vi "NAVX.vi"() -> ()   [LabVIEW 2018]
uses:
  <vilib>/Studica/Studica Toolkit/Background/I2C Channel.ctl
  <vilib>/Studica/Studica Toolkit/NavX/TypeDefs/Flags/Z900_navX_Flags_OpStatusTypeDef.ctl
  <vilib>/Studica/Studica Toolkit/NavX/TypeDefs/Flags/Z900_navX_Flags_CalibrationStatusTypeDef.ctl
  Underlying VI's/NavX VI/navX type def.ctl
  <vilib>/Studica/Studica Toolkit/NavX/NavX.lvlib
panel:
  out "min value":dbl
  out "max value":dbl
  out "Error Out":errorcluster
  out "Status":T3 {"OP Status" items=["INITIALIZING", "SELFTEST_IN_PROGRESS", "ERROR", "IMU_AUTOCAL_IN_PROGRESS", "NORMAL"]; "Calibration Status" items=["IMU_CAL_STATE_MASK"=3, "IMU_CAL_STATE_INPROGRESS"=0, "IMU_CAL_STATE_ACCUMULATE"=1, "IMU_CAL_STATE_COMPLETE"=2]}
  out "NavX Readings":T4
  out "NavX Info Out":T6
  in  "stop":bool
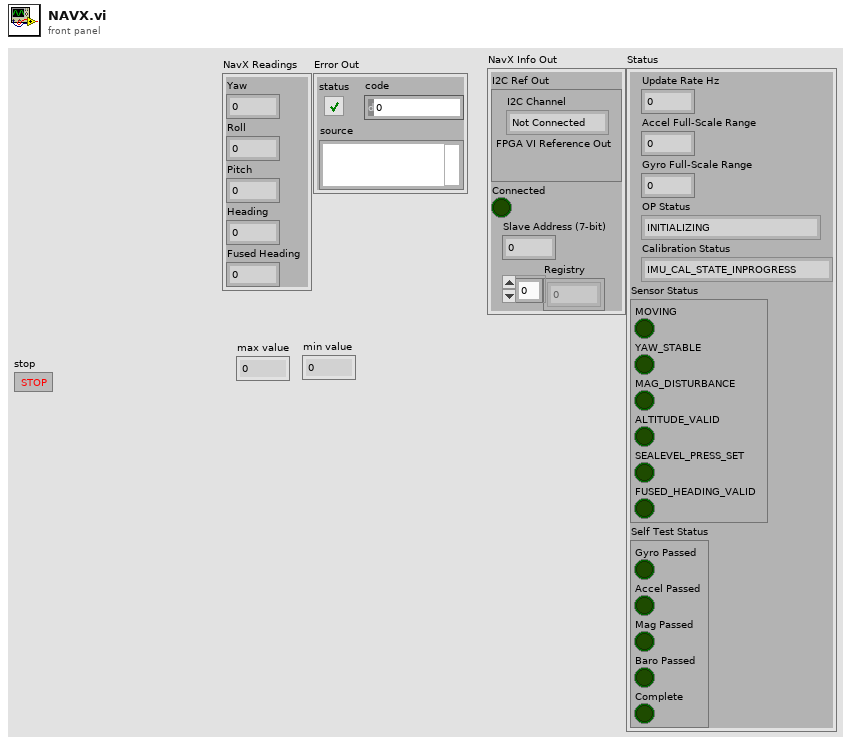
[diagram p1: front panel]
types:
  T1 = typedef "NavX.lvlib/Z900_navX_Flags_OpStatusTypeDef.ctl" = u8
  T2 = typedef "NavX.lvlib/Z900_navX_Flags_CalibrationStatusTypeDef.ctl" = u8
  T3 = cluster{"Update Rate Hz":u8, "Accel Full-Scale Range":u8, "Gyro Full-Scale Range":u16, "OP Status":T1, "Calibration Status":T2, "Sensor Status":cluster{"MOVING":bool, "YAW_STABLE":bool, "MAG_DISTURBANCE":bool, "ALTITUDE_VALID":bool, "SEALEVEL_PRESS_SET":bool, "FUSED_HEADING_VALID":bool}, "Self Test Status":cluster{"Gyro Passed":bool, "Accel Passed":bool, "Mag Passed":bool, "Baro Passed":bool, "Complete":bool}}
  T4 = cluster{"Yaw":dbl, "Roll":dbl, "Pitch":dbl, "Heading":dbl, "Fused Heading":dbl}
  T5 = typedef "I2C Channel.ctl" = enum16{"Not Connected", "A", "B"}
  T6 = cluster{"I2C Ref Out":cluster{"I2C Channel":T5, "FPGA VI Reference Out":refnum<k20>}, "Connected":bool, "Slave Address (7-bit)":u8, "Registry":u8[]}
  T7 = typedef "navX type def.ctl" = enum16{"Get i2C reference", "Read Values", "Zero Yaw"}
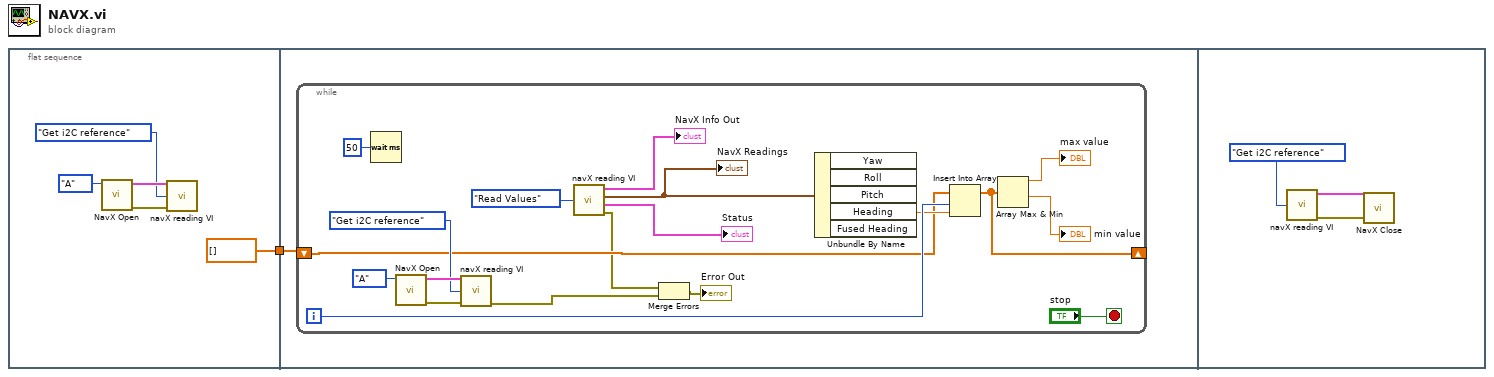
[diagram p0: block diagram]
diagram:
  n1 = flat-sequence {
    tunnel: [dbl[] []] -> w1
    tunnel: w1 -> [w7]
    frame #0 {
      n2 = call <vilib>:"NavX Open.vi"("I2C Channel"=I2C_Channel."A") -> ("error out"=w3:errorcluster, "NavX Info"=w5:T6)  [unwired: 9 in]
      n3 = call "navX reading VI.vi"("NavX Info In"=w5, "Mode"=navX_type_def."Get i2C reference", "error in (no error)"=w3) -> ()  [unwired: 4 out]
    }
    frame #1 {
      n4 = while {
        shift-right: [w11] -> _
        shift-left: w7 -> [w12]
        i -> [w14]
        stop <- "stop" stop-if-true
        n5 = Wait (ms)(milliseconds to wait=u32 50) -> ()  [unwired: 1 out]
        n6 = call <vilib>:"NavX Open.vi"("I2C Channel"=I2C_Channel."A") -> ("error out"=w18:errorcluster, "NavX Info"=w20:T6)  [unwired: 9 in]
        n7 = call "navX reading VI.vi"("NavX Info In"=w20, "Mode"=navX_type_def."Get i2C reference", "error in (no error)"=w18) -> ("Error Out"=w10:errorcluster)  [unwired: 3 out]
        n8 = call "navX reading VI.vi"("Mode"=navX_type_def."Read Values") -> ("NavX Info Out"=→"NavX Info Out":T6, "NavX Readings"=w17:T4, "Status"=→"Status":T3, "Error Out"=w8:errorcluster)  [unwired: 2 in]
        "NavX Readings" <- w17
        n9 = Merge Errors(w8, w10) -> (→"Error Out":errorcluster)
        n10 = Unbundle By Name(w17) -> ("Heading"=w13:dbl)  [unwired: 4 out]
        n11 = Insert Into Array(array=w12, index=w14, new element=w13) -> (w11:dbl[])
        n12 = Array Max & Min(array=w11) -> (max value=→"max value":dbl, min value=→"min value":dbl)  [unwired: 2 out]
      }
    }
    frame #2 {
      n13 = call "navX reading VI.vi"("Mode"=navX_type_def."Get i2C reference") -> ("NavX Info Out"=w28:T6, "Error Out"=w27:errorcluster)  [unwired: 2 in, 2 out]
      n14 = call <vilib>:"NavX Close.vi"("error in (no error)"=w27, "NavX Info In"=w28) -> ()  [unwired: 9 in, 1 out]
    }
  }
